vi "MUX_1BIT.vi"(1 "S":bool, 2 "A2":bool, 3 "A1":bool) -> (0 "Z":bool)   [LabVIEW 2018]
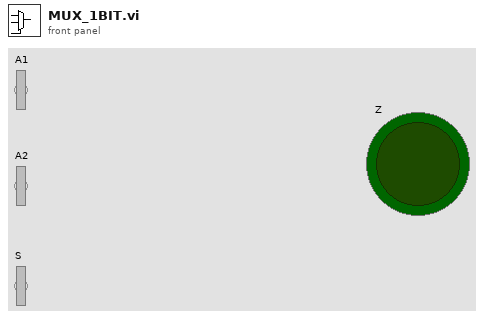
[diagram p1: front panel]
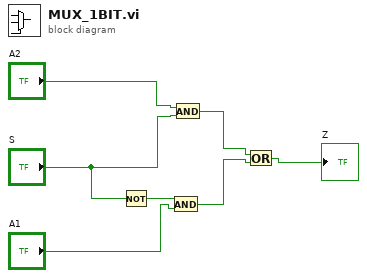
[diagram p0: block diagram]
diagram:
  n1 = Not(x="S") -> (.not. x?=w7:bool)
  n2 = And(x=w7, y="A1") -> (x .and. y?=w3:bool)
  n3 = And(x="A2", y="S") -> (x .and. y?=w2:bool)
  n4 = Or(x=w2, y=w3) -> (x .or. y?=→"Z":bool)
